vi "Agilent_33220A_FuncGen_Serial.vi"() -> ()   [LabVIEW 2019, in "Models of External Instruments.lvlib"]
uses:
  Models of External Instruments.lvlib
  <vilib>/measure/NI_MABase.lvlib
panel:
  out "Numeric":i32
  in  "Stop":bool
  out "error out":errorcluster
  out "read buffer 2":string
  out "Waveform Graph":waveform(dbl)(graph)
  in  "Tab Control":enum32{"SIN", "PULSE", "RAMP", "DC"}(tab)
  in  "SIN Offset":dbl
  in  "SIN Amplitude":dbl
  in  "SIN Frequency":dbl
  in  "PULSE Frequency":dbl
  in  "PULSE Amplitude":dbl
  in  "PULSE Offset":dbl
  in  "RAMP Frequency":dbl
  in  "RAMP Amplitude":dbl
  in  "RAMP Offset":dbl
  in  "DC Amplitude":dbl
  in  "DC Frequency":dbl
  in  "DC Offset":dbl
  out "read buffer":string
  out "Vpp":string
  out "Offset":string
  out "Waveform Type":string
  out "Frequency":string
  in  "Output On/OFF":bool
  out "Read Error Out":errorcluster
  out "Write Error Out":errorcluster
  out "Result Waveform":string
  in  "VISA Open timeout (0)":u32
  # "Output Configuration Commands\n\nOUTP ON\nOUTP OFF \n\nOUTP? --> 1 ON, 0 OFF\n\nOUTP:LOAD? -->yük empedansı\nOUTP:LOAD?  MAX--> maks yük empedansı\nOUTP:LOAD?  MIN--> min yük empedansı\n\nOUTP:POL? --> Normal or Inverted\nOUTP:POL INV -->Inverted waveform\nOUTP:POL?\n\nOUTP:POL NORM-->Normal Waveform\nOUTP:POL?\n\nOUTP:SYNC ON  -->Sync konnectörünü aktif eder\nOUTP:SYNC OFF -->Sync konnectörünü deaktif eder\nOUTP:SYNC? --> Sync konnectörünün durumu 1-ON, 0-OFF\n\nVOLT:UNIT? --> Voltaj biriminin durumu\nVOLT:UNIT VRMS -->birim Vrms\nVOLT:UNIT VPP -->birim Vpp\nVOLT:UNIT DBM -->birim dBm"
  # "Pulse Configuration Commands\n\nPULS:PER 5  --> saniye cinsinden darbe periydunun ayarı\nPULS:PER MIN --> Minimumu 200ns olarak ayarlar\nPULS:PER MAX --> Maxı 2000s olarak ayarlar\nPULS:PER? -*->pulse periyot durumu\n\nFUNC:PULSE:HOLD WID --> pulse genişliği şeklinde ayarla\nFUNC:PULSE:HOLD DCYC --> pulse duty cycle şeklinde ayarla\nFUNC:PULSE:HOLD -->Pulse ayar durumu\n\nFUNC:PULS:WIDT 5-->Pulse genişliği saniye cinsinden ayarla\nFUNC:PULS:WIDT MAX --> Pulse genişliğini max 1999.99 s olarak ayarla\nFUNC:PULS:WIDT MIN --> Pulse genişliğini min 20ns olarak ayarla\nFUNC:PULS:WIDT? --> Pulse genişliğinin durumu\n\nFUNC:PULS:DCYC 50-->Pulse duty cycle'ını oran cinsinden ayarla\nFUNC:PULS:DCYC MAX -->Pulse duty cycle'ını max 100% olarak ayarla\nFUNC:PULS:DCYC MIN --> Pulse duty cycle'ını  min 0% olarak ayarla\nFUNC:PULS:DCYC? -->  Pulse duty cycle'ının durumu\n\nFUNC:PULS:TRAN 50 --> düşen ve yükselen kenar için edge time'ı oran olarak ayarla\n                                             edge time from 5 ns to 100 ns\nFUNC:PULS:TRAN MAX --> edge time 100ns\nFUNC:PULS:TRAN MIN --> edge time 5ns\nFUNC:PULS:TRAN? -->edge time durumu"
  # "APPLy Command\n\nAPPL:SIN 5 KHZ, 3.0 VPP, -2.5 V\nAPPL?\n\nAPPL:SIN 5.0E+3, 3.0 VRMS, -2.5\nAPPL?\n\nAPPL:SQU 5.0E+3, 3.0, -2.5\nAPPL?"
  # "APPLy\n:SINusoid [<frequency> [,<amplitude> [,<offset>] ]]\n:SQUare [<frequency> [,<amplitude> [,<offset>] ]]\n:RAMP [<frequency> [,<amplitude> [,<offset>] ]]\n:PULSe [<frequency> [,<amplitude> [,<offset>] ]]\n:NOISe [<frequency|DEF>1 [,<amplitude> [,<offset>] ]]\n:DC [<frequency|DEF>1 [,<amplitude>|DEF>1 [,<offset>] ]]\n:USER [<frequency> [,<amplitude> [,<offset>] ]]\nAPPLy?"
  # "Low-Level Commands\n\nFUNC SIN --> Select sine wave function\nFREQ 5000 -->Set frequency to 5 kHz\nVOLT 3.0 --> Set amplitude to 3 Vpp\nVOLT:OFFS -2.5 --> Set offset to -2.5 Vdc\nAPPL?"
  # "*IDN? --> cihaz bilgileri: Agilent Technologies,33220A,<serial number>,f.ff-b.bb-aa-p\n                                            f.ff = Firmware revision number\n                                            b.bb = Boot kernel revision number\n                                            aa = ASIC revision number\n                                            p = Printed circuit board revision number\nSYSTem:VERSion? --> sistem verisyonu\n\nSYST:ERR? --> Hataları oku\n\nDISP ON--> ekranı aç\nDISP OFF--> ekranı kapat\nDISP? --> ekran durumu"
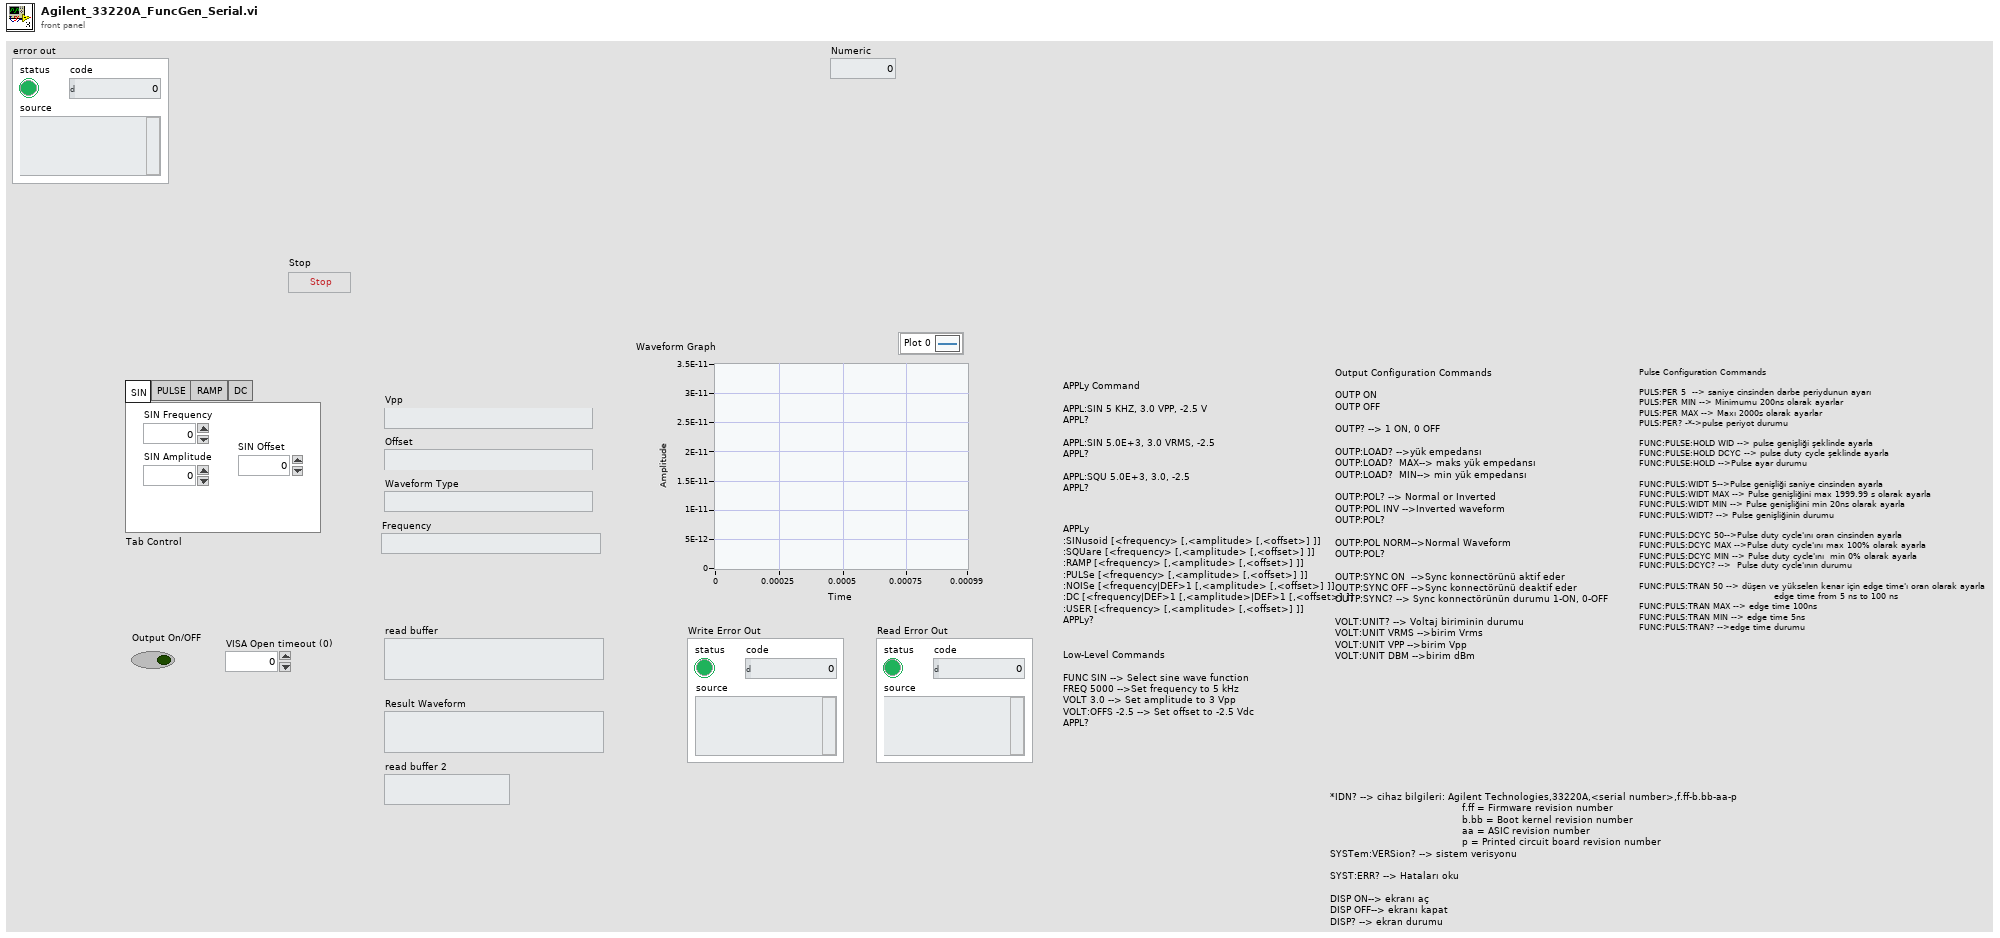
[diagram p1: front panel]
types:
  T1 = enum16{"Sine Wave", "Triangle Wave", "Square Wave", "Sawtooth Wave"}
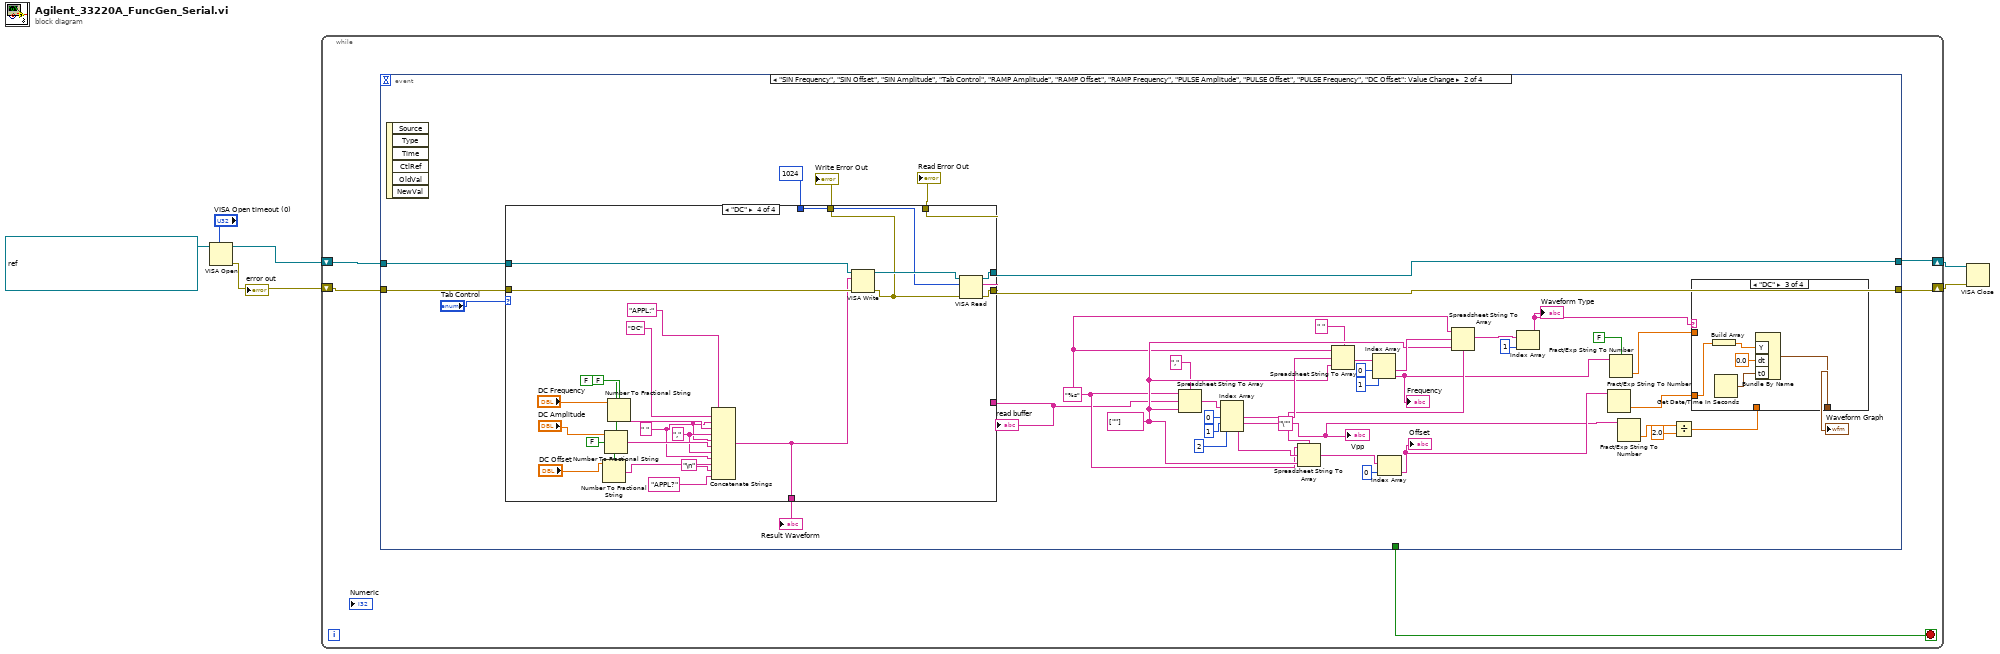
[diagram p0: block diagram]
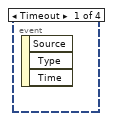
[diagram p2: hidden frame]
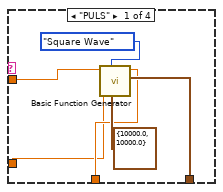
[diagram p3: hidden frame]
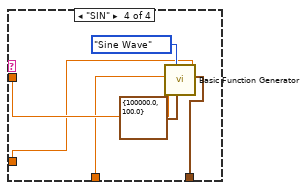
[diagram p5: hidden frame]
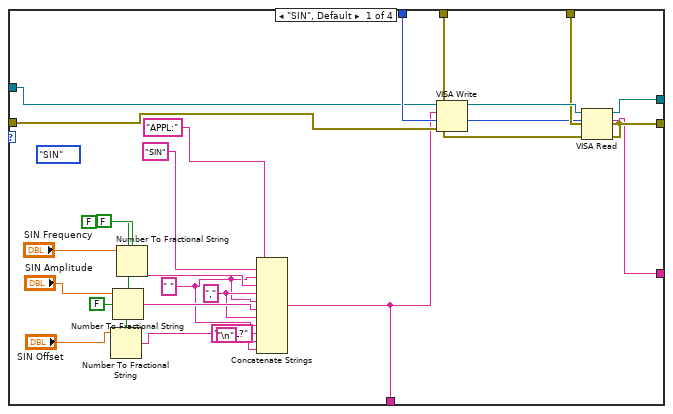
[diagram p6: hidden frame]
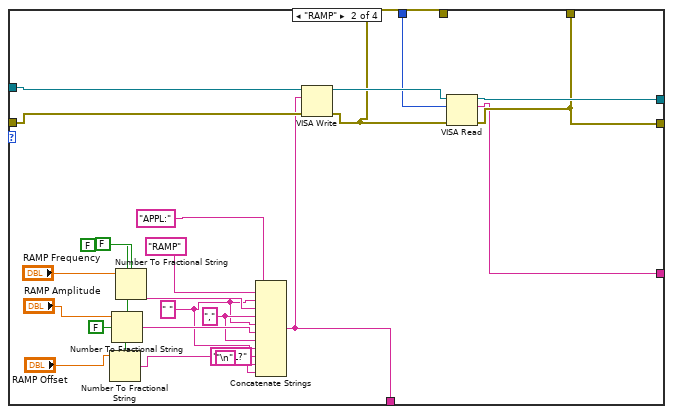
[diagram p7: hidden frame]
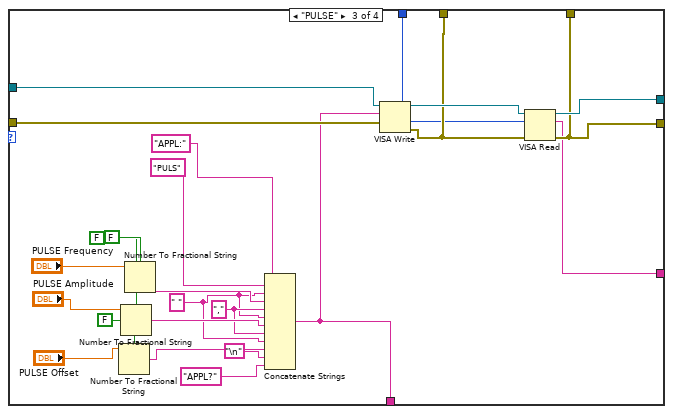
[diagram p8: hidden frame]
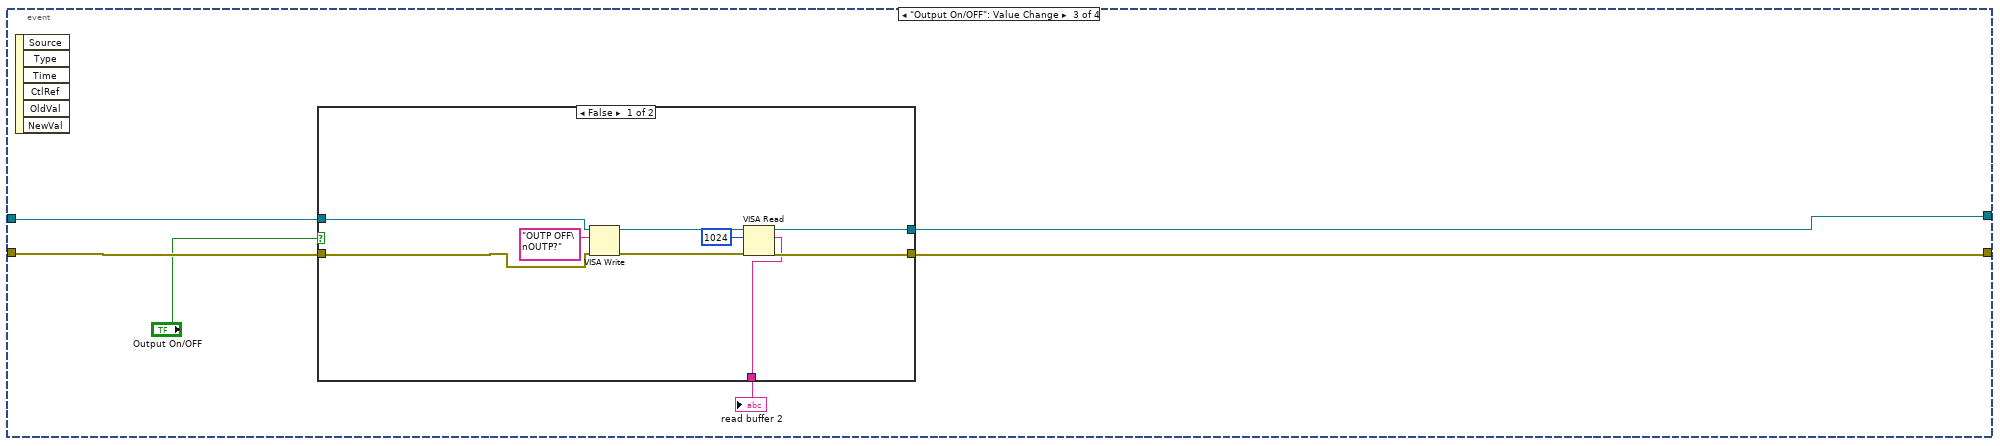
[diagram p9: hidden frame]
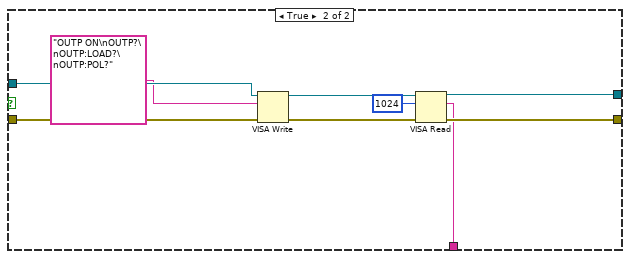
[diagram p10: hidden frame]
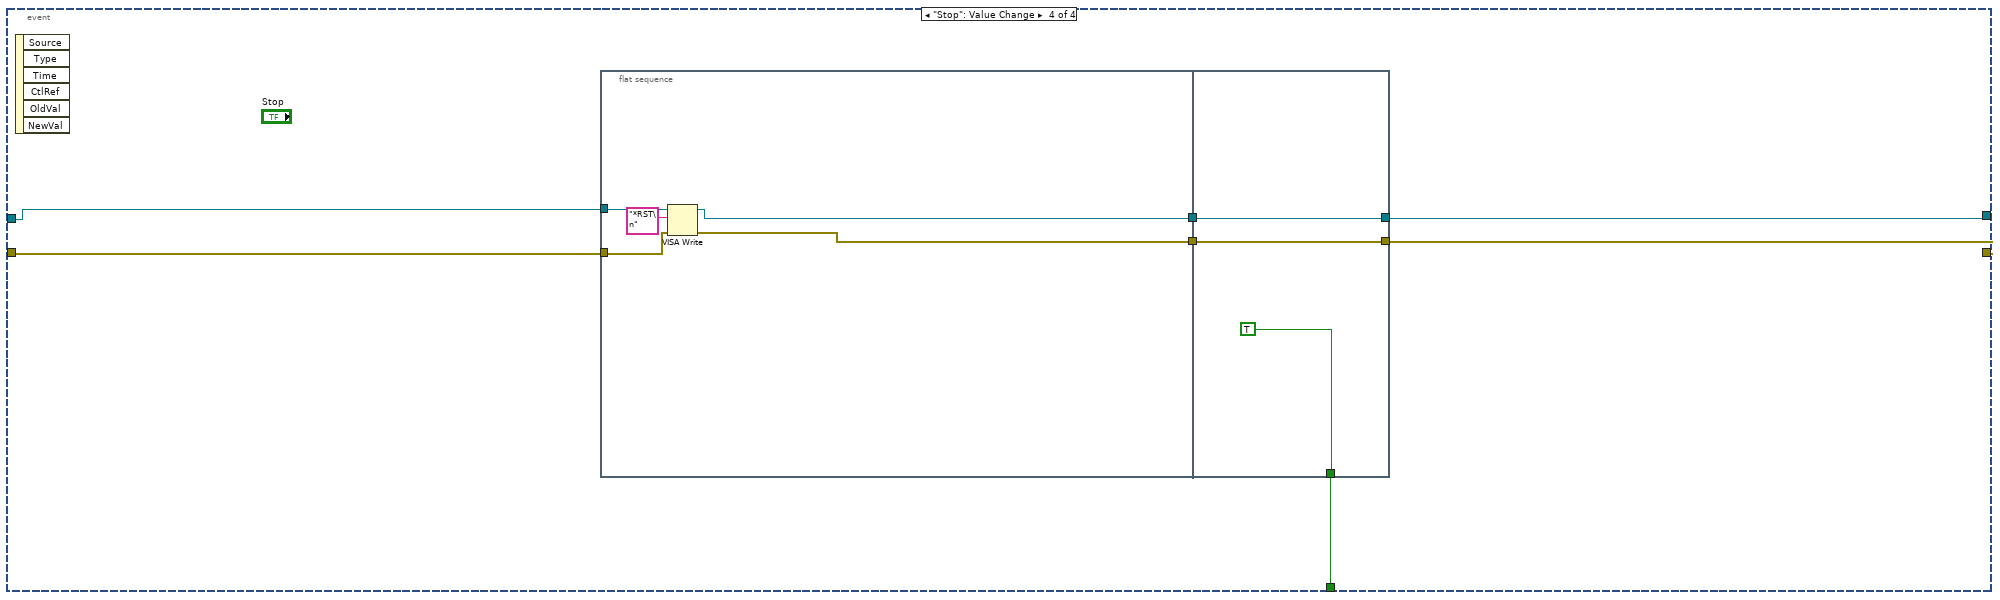
[diagram p11: hidden frame]
diagram:
  n1 = VISA Open(timeout (0)="VISA Open timeout (0)", VISA resource name=refnum<visa-resource-name> "TCPIP0::10.41.74.80::inst0::INSTR") -> (VISA resource name=w1:refnum<visa-resource-name>, error out=w6:errorcluster)  [unwired: 3 in]
  "error out" <- w6
  n2 = while {
    shift-right: [w10] -> w3
    shift-left: w6 -> [w11]
    shift-right: [w9] -> w2
    shift-left: w1 -> [w8]
    stop <- w7 stop-if-true
    n3 = event shown="[1] \"SIN Frequency\", \"SIN Offset\", \"SIN Amplitude\", \"Tab Control\", \"RAMP Amplitude\", \"RAMP Offset\", \"RAMP Frequency\", \"PULSE Amplitude\", \"PULSE Offset\", \"PULSE Frequency\", \"DC Offset\": Value Change" {
      selector: _ -> [_ _ _ _]
      dyn-events: _ -> [_ _ _ _]
      timeout: _ -> [_ _ _ _]
      tunnel: w11 -> [_ w49 w170 w194]
      tunnel: [_ w51 w169 w193] -> w9
      tunnel: [_ w50 w168 w192] -> w10
      tunnel: w8 -> [_ w18 w165 w195]
      tunnel: [_ _ _ w189] -> w7
      event Timeout {
        n4 = event-data() -> ()  [unwired: 1 in, 3 out]
      }
      event "SIN Frequency", "SIN Offset", "SIN Amplitude", "Tab Control", "RAMP Amplitude", "RAMP Offset", "RAMP Frequency", "PULSE Amplitude", "PULSE Offset", "PULSE Frequency", "DC Offset": Value Change {
        w36 = "\"" ("delimiter (Tab)")
        w35 = string[] [""]
        w34 = "%s" ("format string")
        n5 = event-data() -> ()  [unwired: 1 in, 6 out]
        n6 = case shown="\"DC\"" "Tab Control" {
          tunnel: [w88 w115 w139 w163] -> w51
          tunnel: [w78 w113 w137 w161] -> w50
          tunnel: [w79 w114 w138 w162] -> w48
          tunnel: [w78 w113 w137 w161] -> w47
          tunnel: w49 -> [w73 w112 w136 w160]
          tunnel: u32 1024 ("byte count") -> [w72 w111 w135 w159]
          tunnel: [w71 w110 w134 w158] -> w24
          tunnel: [w70 w94 w118 w141] -> w19
          tunnel: w18 -> [w69 w93 w117 w142]
          frame "SIN", Default {
            w77 = " " ("string")
            (unwired) enum32{"SIN", "PULSE", "RAMP", "DC"}."SIN" ("Tab Control")
            w82 = "," ("string")
            n7 = Number To Fractional String(use system decimal point (T)=FALSE, number="SIN Offset") -> (F-format string=w89:string)  [unwired: 2 in]
            n8 = Number To Fractional String(use system decimal point (T)=FALSE, number="SIN Amplitude") -> (F-format string=w87:string)  [unwired: 2 in]
            n9 = Number To Fractional String(use system decimal point (T)=FALSE, number="SIN Frequency") -> (F-format string=w85:string)  [unwired: 2 in]
            n10 = Concatenate Strings("APPL:", "SIN", w77, w85, w82, w77, w87, w82, w77, w89, "\n", "APPL?" ("string")) -> (w70:string)
            n11 = VISA Write(VISA resource name=w69, write buffer=w70, error in (no error)=w73) -> (VISA resource name out=w92:refnum<visa-resource-name>, error out=w79:errorcluster)  [unwired: 1 out]
            n12 = VISA Read(VISA resource name=w92, byte count=w72, error in (no error)=w79) -> (VISA resource name out=w88:refnum<visa-resource-name>, read buffer=w71:string, error out=w78:errorcluster)  [unwired: 1 out]
          }
          frame "RAMP" {
            w99 = " " ("string")
            w102 = "," ("string")
            n13 = Number To Fractional String(use system decimal point (T)=FALSE, number="RAMP Offset") -> (F-format string=w107:string)  [unwired: 2 in]
            n14 = Number To Fractional String(use system decimal point (T)=FALSE, number="RAMP Amplitude") -> (F-format string=w106:string)  [unwired: 2 in]
            n15 = Number To Fractional String(use system decimal point (T)=FALSE, number="RAMP Frequency") -> (F-format string=w104:string)  [unwired: 2 in]
            n16 = Concatenate Strings("APPL:", "RAMP", w99, w104, w102, w99, w106, w102, w99, w107, "\n", "APPL?" ("string")) -> (w94:string)
            n17 = VISA Write(VISA resource name=w93, write buffer=w94, error in (no error)=w112) -> (VISA resource name out=w116:refnum<visa-resource-name>, error out=w114:errorcluster)  [unwired: 1 out]
            n18 = VISA Read(VISA resource name=w116, byte count=w111, error in (no error)=w114) -> (VISA resource name out=w115:refnum<visa-resource-name>, read buffer=w110:string, error out=w113:errorcluster)  [unwired: 1 out]
          }
          frame "PULSE" {
            w123 = " " ("string")
            w126 = "," ("string")
            n19 = Number To Fractional String(use system decimal point (T)=FALSE, number="PULSE Offset") -> (F-format string=w131:string)  [unwired: 2 in]
            n20 = Number To Fractional String(use system decimal point (T)=FALSE, number="PULSE Amplitude") -> (F-format string=w130:string)  [unwired: 2 in]
            n21 = Number To Fractional String(use system decimal point (T)=FALSE, number="PULSE Frequency") -> (F-format string=w128:string)  [unwired: 2 in]
            n22 = Concatenate Strings("APPL:", "PULS", w123, w128, w126, w123, w130, w126, w123, w131, "\n", "APPL?" ("string")) -> (w118:string)
            n23 = VISA Write(VISA resource name=w117, write buffer=w118, error in (no error)=w136) -> (VISA resource name out=w140:refnum<visa-resource-name>, error out=w138:errorcluster)  [unwired: 1 out]
            n24 = VISA Read(VISA resource name=w140, byte count=w135, error in (no error)=w138) -> (VISA resource name out=w139:refnum<visa-resource-name>, read buffer=w134:string, error out=w137:errorcluster)  [unwired: 1 out]
          }
          frame "DC" {
            w147 = " " ("string")
            w150 = "," ("string")
            n25 = Number To Fractional String(use system decimal point (T)=FALSE, number="DC Offset") -> (F-format string=w155:string)  [unwired: 2 in]
            n26 = Number To Fractional String(use system decimal point (T)=FALSE, number="DC Amplitude") -> (F-format string=w154:string)  [unwired: 2 in]
            n27 = Number To Fractional String(use system decimal point (T)=FALSE, number="DC Frequency") -> (F-format string=w152:string)  [unwired: 2 in]
            n28 = Concatenate Strings("APPL:", "DC", w147, w152, w150, w147, w154, w150, w147, w155, "\n", "APPL?" ("string")) -> (w141:string)
            n29 = VISA Write(VISA resource name=w142, write buffer=w141, error in (no error)=w160) -> (VISA resource name out=w164:refnum<visa-resource-name>, error out=w162:errorcluster)  [unwired: 1 out]
            n30 = VISA Read(VISA resource name=w164, byte count=w159, error in (no error)=w162) -> (VISA resource name out=w163:refnum<visa-resource-name>, read buffer=w158:string, error out=w161:errorcluster)  [unwired: 1 out]
          }
        }
        "read buffer" <- w24
        "Result Waveform" <- w19
        "Write Error Out" <- w48
        "Read Error Out" <- w47
        n31 = Spreadsheet String To Array(delimiter (Tab)=",", format string=w34, spreadsheet string=w24, array type (2D Dbl)=w35) -> (array=w37:string[])
        n32 = Index Array(array=w37, index #1=0 ("index"), index #2=1 ("index"), index #3=2 ("index")) -> (element #1=w38:string, element #2=w22:string, element #3=w40:string)
        "Vpp" <- w22
        n33 = Spreadsheet String To Array(delimiter (Tab)=w36, format string=w34, spreadsheet string=w40, array type (2D Dbl)=w35) -> (array=w41:string[])
        n34 = Spreadsheet String To Array(delimiter (Tab)=" ", format string=w34, spreadsheet string=w38, array type (2D Dbl)=w35) -> (array=w39:string[])
        n35 = Index Array(array=w39, index #1=0 ("index"), index #2=1 ("index")) -> (element #1=w42:string, element #2=w21:string)
        "Frequency" <- w21
        n36 = Index Array(array=w41, index=0) -> (element=w23:string)
        "Offset" <- w23
        n37 = Spreadsheet String To Array(delimiter (Tab)=w36, format string=w34, spreadsheet string=w42, array type (2D Dbl)=w35) -> (array=w43:string[])
        n38 = Index Array(array=w43, index=1) -> (element=w20:string)
        "Waveform Type" <- w20
        n39 = Fract/Exp String To Number(string=w23) -> (number=w12:dbl)  [unwired: 3 in, 1 out]
        n40 = Fract/Exp String To Number(use system decimal point (T)=FALSE, string=w21) -> (number=w14:dbl)  [unwired: 2 in, 1 out]
        n41 = Fract/Exp String To Number(string=w22) -> (number=w15:dbl)  [unwired: 3 in, 1 out]
        n42 = Divide(x=w15, y=2.0) -> (x/y=w13:dbl)
        n43 = case shown="\"DC\"" w20 {
          tunnel: [w56 _ w61 w67] -> w16
          tunnel: w14 -> [w54 _ _ w66]
          tunnel: w13 -> [w53 _ _ w64]
          tunnel: w12 -> [w52 _ w58 w65]
          frame "PULS" {
            n44 = call <vilib>:"Basic Function Generator.vi"("offset"=w53, "sampling info"=cluster{"Fs":dbl, "#s":dbl} {"Fs"=10000.0, "#s"=10000.0}, "signal type"=T1."Square Wave", "amplitude"=w52, "frequency"=w54) -> ("signal out"=w56:waveform(dbl))  [unwired: 4 in, 2 out]
          }
          frame Default {
          }
          frame "DC" {
            n45 = Build Array(w58) -> (w62:dbl[])
            n46 = Get Date/Time In Seconds() -> (seconds since 1Jan1904=w59:timestamp)
            n47 = Bundle By Name("Y"=w62, "dt"=0.0, "t0"=w59) -> (w61:waveform(dbl))  [unwired: 1 in]
          }
          frame "SIN" {
            n48 = call <vilib>:"Basic Function Generator.vi"("offset"=w65, "sampling info"=cluster{"Fs":dbl, "#s":dbl} {"Fs"=100000.0, "#s"=100.0}, "signal type"=T1."Sine Wave", "amplitude"=w64, "frequency"=w66) -> ("signal out"=w67:waveform(dbl))  [unwired: 4 in, 2 out]
          }
        }
        "Waveform Graph" <- w16
      }
      event "Output On/OFF": Value Change {
        n49 = event-data() -> ()  [unwired: 1 in, 6 out]
        n50 = case shown="False" "Output On/OFF" {
          tunnel: w170 -> [w173 w188]
          tunnel: [w176 w185] -> w169
          tunnel: [w175 w184] -> w168
          tunnel: [w174 w183] -> w166
          tunnel: w165 -> [w171 w181]
          frame False {
            n51 = VISA Write(VISA resource name=w171, write buffer="OUTP OFF\nOUTP?", error in (no error)=w173) -> (VISA resource name out=w178:refnum<visa-resource-name>, error out=w177:errorcluster)  [unwired: 1 out]
            n52 = VISA Read(VISA resource name=w178, byte count=u32 1024, error in (no error)=w177) -> (VISA resource name out=w176:refnum<visa-resource-name>, read buffer=w174:string, error out=w175:errorcluster)  [unwired: 1 out]
          }
          frame True {
            n53 = VISA Write(VISA resource name=w181, write buffer="OUTP ON\nOUTP?\nOUTP:LOAD?\nOUTP:POL?", error in (no error)=w188) -> (VISA resource name out=w187:refnum<visa-resource-name>, error out=w186:errorcluster)  [unwired: 1 out]
            n54 = VISA Read(VISA resource name=w187, byte count=u32 1024, error in (no error)=w186) -> (VISA resource name out=w185:refnum<visa-resource-name>, read buffer=w183:string, error out=w184:errorcluster)  [unwired: 1 out]
          }
        }
        "read buffer 2" <- w166
      }
      event "Stop": Value Change {
        n55 = event-data() -> ()  [unwired: 1 in, 6 out]
        n56 = flat-sequence {
          tunnel: w195 -> [w200]
          tunnel: w194 -> [w199]
          tunnel: [w196] -> w191
          tunnel: [w197] -> w190
          tunnel: [w202] -> w192
          tunnel: [w203] -> w193
          tunnel: w191 -> [w203]
          tunnel: w190 -> [w202]
          tunnel: [TRUE] -> w189
          frame #0 {
            n57 = VISA Write(VISA resource name=w200, write buffer="*RST\n", error in (no error)=w199) -> (VISA resource name out=w196:refnum<visa-resource-name>, error out=w197:errorcluster)  [unwired: 1 out]
          }
          frame #1 {
          }
        }
      }
    }
  }
  n58 = VISA Close(VISA resource name=w2, error in (no error)=w3) -> ()  [unwired: 1 out]
